vi "User - Edit.vi"(0 "VISA resource name":refnum<visa-resource-name>, 1 "User Pointer(1-299)":i32=1, 2 "User Name (8 character max)":string, 3 "Password (8 number max)":string, 4 "Level":u16(ring)=1 items=["Run Only", "Recall Setup", "Edit Step", "Full System"], 5 "error in (no error)":errorcluster) -> (14 "VISA resource name out":refnum<visa-resource-name>, 19 "error out":errorcluster)   [LabVIEW 2020, in "eec EST 300.lvlib"]
doc: "Edit user\n1.User Pointer\n2.User ID\n3.Password\n4.Security Level:\n 0=Run Only: This is the most restricted mode of user access. You can only initiate a test, reset a failure or abort a test from the Perform Tests screen.\n\n 1=Recall Setup: This mode allows you to load previously configured test files but it does not allow any editing of the parameters. In this mode you are restricted from access to the “Setup Test Parameters” screen.\n\n 2=Edit Step: In this mode you can load files and edit test parameters.\n\n 3=Full System: In this mode you have full access level to all instrument setup parameters as well as system configuration and security levels. Access at this level should be restricted to System Administrators."
uses:
  <instrlib>/eec EST 300/eec EST 300.lvlib
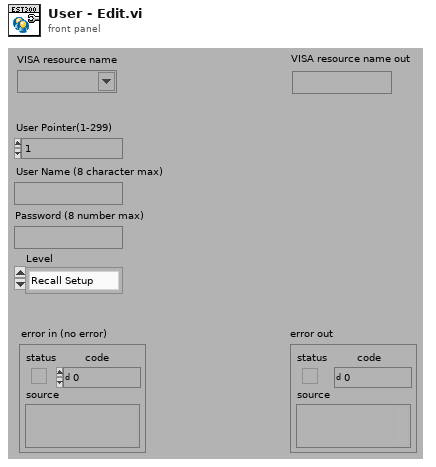
[diagram p1: front panel]
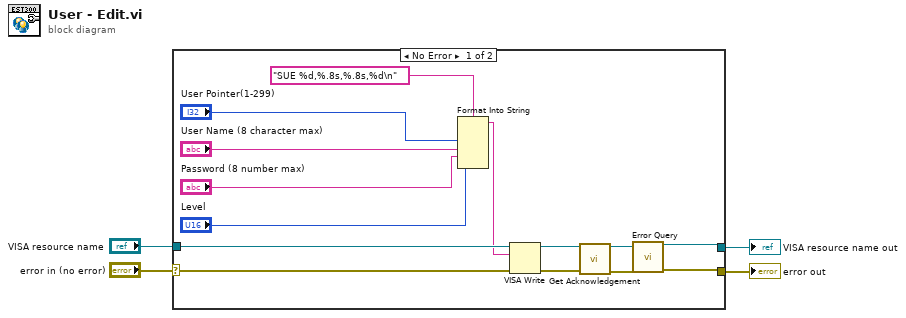
[diagram p0: block diagram]
diagram:
  n1 = case shown="No Error" "error in (no error)" {
    selector: "error in (no error)" -> [w7 w19]
    tunnel: "VISA resource name" -> [w9 w20]
    tunnel: [w6 w20] -> w3
    tunnel: [w5 w19] -> w2
    frame No Error {
      n2 = Format Into String(format string="SUE %d,%.8s,%.8s,%d\n" ("\"False\" Command"), "User Pointer(1-299)", "User Name (8 character max)", "Password (8 number max)", "Level") -> (resulting string=w8:string)  [unwired: 2 in, 1 out]
      n3 = VISA Write(VISA resource name=w9, write buffer=w8, error in (no error)=w7) -> (VISA resource name out=w11:refnum<visa-resource-name>, error out=w10:errorcluster)  [unwired: 1 out]
      n4 = call <instrlib>:"Get Acknowledgement.vi"("VISA resource name"=w11, "error in (no error)"=w10) -> ("VISA resource name out"=w13:refnum<visa-resource-name>, "error out"=w12:errorcluster)  [unwired: 12 in]
      n5 = call <instrlib>:"Error Query.vi"("VISA resource name"=w13, "error in (no error)"=w12) -> ("VISA resource name out"=w6:refnum<visa-resource-name>, "error out"=w5:errorcluster)  [unwired: 10 in, 2 out]
    }
    frame Error {
    }
  }
  "error out" <- w2
  "VISA resource name out" <- w3
